vi "Checksum Test.vi"() -> ()   [LabVIEW 2010]
panel:
  out "Numeric":u8 format="%x"
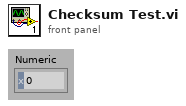
[diagram p1: front panel]
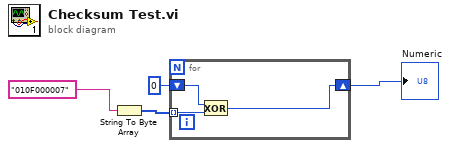
[diagram p0: block diagram]
diagram:
  n1 = String To Byte Array(string="010F000007") -> (unsigned byte array=w3:u8[])
  n2 = for {
    tunnel: w3 -> [w6] mode=indexing
    shift-right: [w7] -> w1
    shift-left: u8 0 -> [w5]
    n3 = Exclusive Or(1:w6, 2:w5) -> (0:w7:u8)
  }
  "Numeric" <- w1
